vi "PXI-2510 Channel Page.vi"(8 "error in (no error)":errorcluster, 11 "Node Ptr":T2 format="%.0x") -> (0 "error out":errorcluster)   [LabVIEW 2011, in "PXI-2510 Custom Device.lvlib"]
uses:
  PXI-2510 Custom Device.lvlib
  <vilib>/NI Veristand/Custom Device API/Custom Device Item Ref.ctl
  Channel Fault Selector.ctl
  FIU Global Strings.vi
  <vilib>/NI Veristand/Custom Device API/Get Item Property (U16).vi
  <vilib>/NI Veristand/Custom Device API/Custom Device API.lvlib
panel:
  out "Hardware Channel #":u16
  in  "Channel Fault Selector Default Value":T1
  in  "Header":cluster{"Section Name":string}={"Section Name"="Custom Device Item Settings"}
  in  "Description":string
  in  "Name (Alias)":string
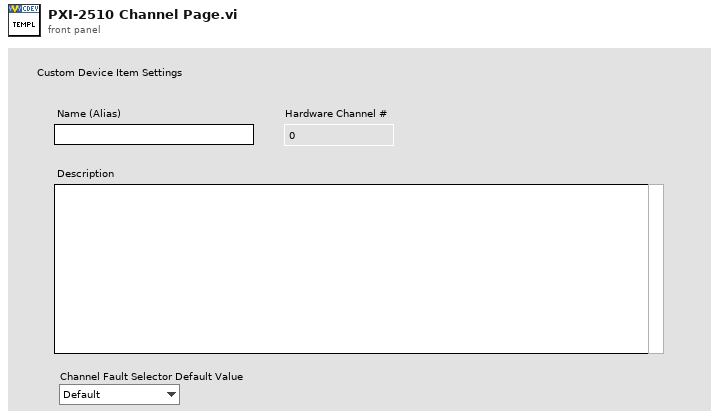
[diagram p1: front panel]
types:
  T1 = typedef "PXI-2510 Custom Device.lvlib/Channel Fault Selector.ctl" = enum16{"Default", "DUT Pass Through", "DUT Open", "DUT Pass Through and FB A", "DUT Pass Through and FB B", "DUT FB A", "DUT FB B"}
  T2 = typedef "Custom Device API.lvlib/Custom Device Item Ref.ctl" = u64
  T3 = typedef "Custom Device API.lvlib/Custom Device Item Info.ctl" = cluster{"Name":string, "Is Channel":bool, "GUID":string}
  T4 = typedef "Custom Device API.lvlib/Custom Device Channel.ctl" = cluster{"Type":T5, "Units":string, "Default Value":dbl, "Faultable":bool, "Scalable":bool}
  T5 = typedef "Custom Device API.lvlib/Custom Device Channel Type.ctl" = enum16{"Input", "Output"}
  T6 = typedef "Custom Device API.lvlib/Custom Device Commands.ctl" = enum16{"Default", "Item renamed", "Shutdown", "Dynamic button pressed"}
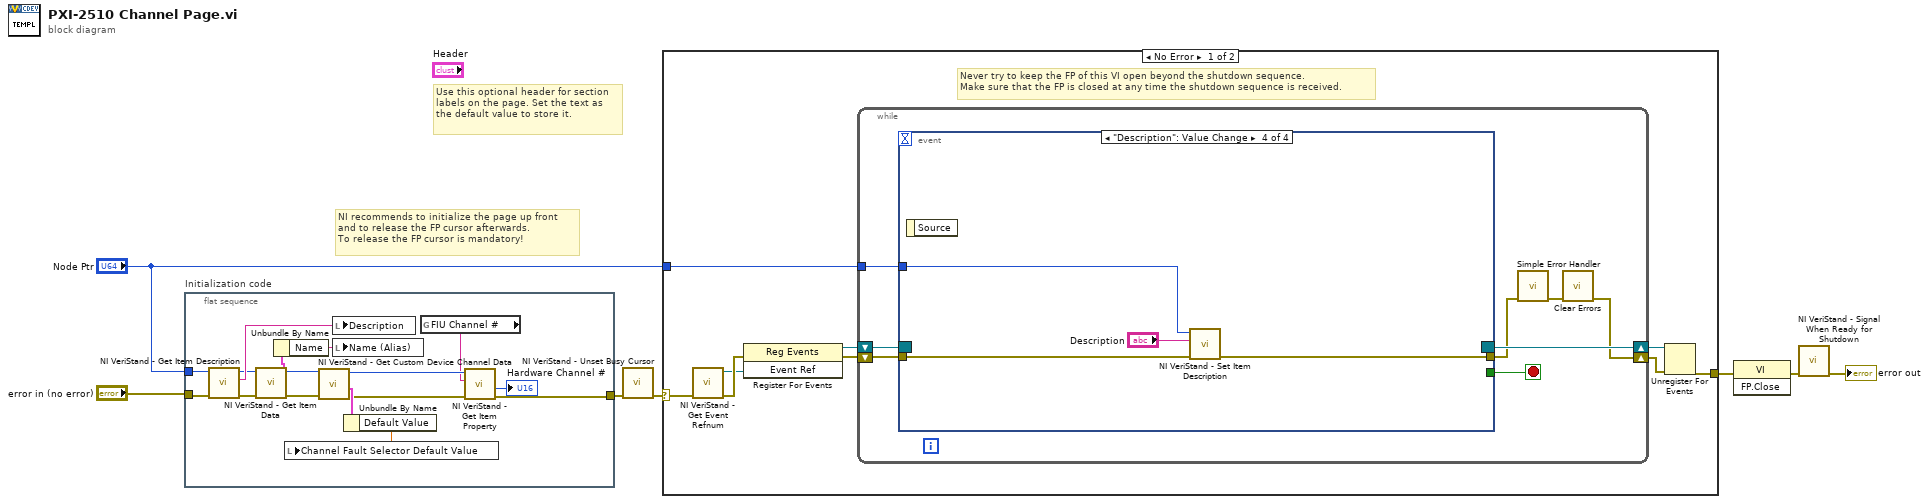
[diagram p0: block diagram]
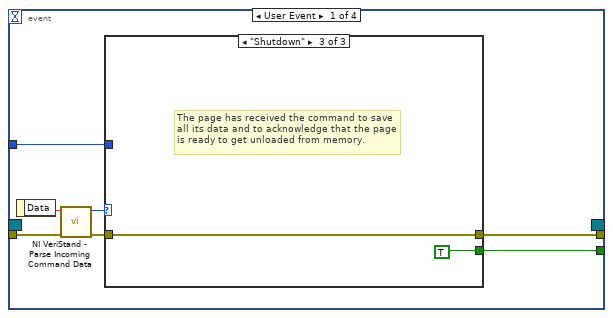
[diagram p2: hidden frame]
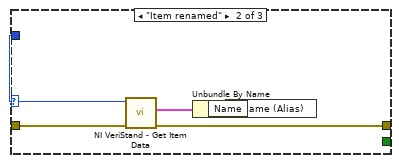
[diagram p4: hidden frame]
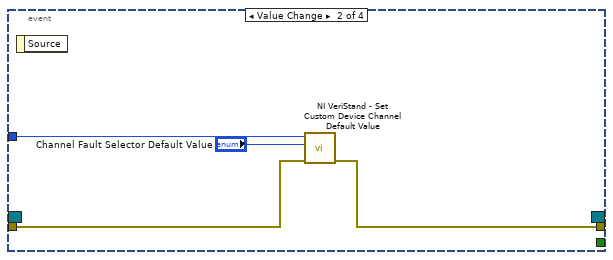
[diagram p5: hidden frame]
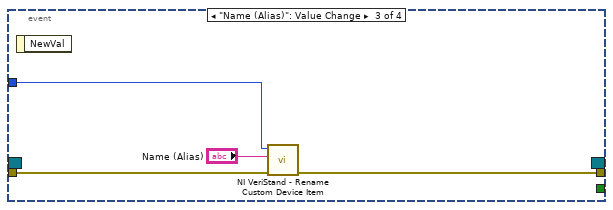
[diagram p6: hidden frame]
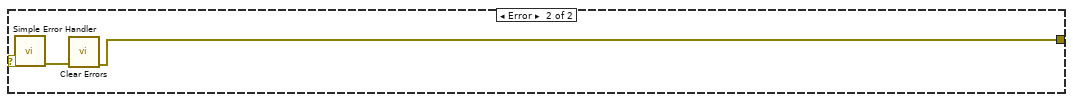
[diagram p7: hidden frame]
diagram:
  # "Use this optional header for section labels on the page. Set the text as the default value to store it."
  # "NI recommends to initialize the page up front\nand to release the FP cursor afterwards.\nTo release the FP cursor is mandatory!"
  n1 = flat-sequence "Initialization code" {
    tunnel: "error in (no error)" -> [w23]
    tunnel: "Node Ptr" -> [w22]
    tunnel: [w8] -> w2
    frame #0 {
      n2 = call <vilib>:"NI VeriStand - Get Item Description.vi"("error in (no error)"=w23, "Item Ref in"=w22) -> ("error out"=w20:errorcluster, "Description"=w21:string, "Item Ref out"=w19:T2)  [unwired: 7 out]
      n3 = call <vilib>:"NI VeriStand - Get Item Data.vi"("error in (no error)"=w20, "Item Ref in"=w19) -> ("error out"=w15:errorcluster, "Item Info"=w18:T3, "Item Ref out"=w16:T2)  [unwired: 7 out]
      n4 = Unbundle By Name(w18) -> ("Name"=w17:string)
      n5 = call <vilib>:"NI VeriStand - Get Custom Device Channel Data.vi"("error in (no error)"=w15, "Channel Ref in"=w16) -> ("error out"=w11:errorcluster, "Channel"=w14:T4, "Channel Ref out"=w12:T2)  [unwired: 4 in, 3 out]
      n6 = local write "Description"(w21) -> ()
      n7 = local write "Name (Alias)"(w17) -> ()
      n8 = Unbundle By Name(w14) -> ("Default Value"=w13:dbl)
      n9 = local write "Channel Fault Selector Default Value"(w13) -> ()
      n10 = global read "FIU Global Strings.vi" "FIU Channel #"() -> (w10:string)
      n11 = call-poly <vilib>:"NI VeriStand - Get Item Property.vi"("error in (no error)"=w11, "Property Name"=w10, "Item Ref in"=w12) -> ("error out"=w8:errorcluster, "Value"=→"Hardware Channel #":u16)  [unwired: 5 in, 2 out]
    }
  }
  n12 = call <vilib>:"NI VeriStand - Unset Busy Cursor.vi"("error in (no error)"=w2) -> ("error out"=w1:errorcluster)  [unwired: 10 out]
  n13 = case shown="No Error" w1 {
    selector: w1 -> [w24 w70]
    tunnel: [w29 w68] -> w5
    tunnel: "Node Ptr" -> [w25 _]
    frame No Error {
      # "Never try to keep the FP of this VI open beyond the shutdown sequence.\nMake sure that the FP is closed at any time the shutdown sequence is received."
      n14 = call <vilib>:"NI VeriStand - Get Event Refnum.vi"("error in (no error)"=w24) -> ("error out"=w32:errorcluster, "Event Ref"=w28:refnum<user-event>)  [unwired: 9 out]
      n15 = register-events(error in=w32, w28) -> (reference out=w26:refnum<event-registration>, error out=w27:errorcluster)  [unwired: 1 in]
      n16 = while {
        tunnel: w25 -> [w36]
        shift-right: [w33] -> w30
        shift-left: w27 -> [w39]
        shift-right: [w40] -> w31
        shift-left: w26 -> [w38]
        stop <- w37 stop-if-true
        n17 = event shown="[3] \"Description\": Value Change" {
          selector: w38 -> [_ _ _ _]
          dyn-events: [_ _ _ _] -> w40
          timeout: _ -> [_ _ _ _]
          tunnel: w39 -> [w47 w57 w63 w66]
          tunnel: [w43 _ _ _] -> w37
          tunnel: [w42 w56 w62 w65] -> w35
          tunnel: w36 -> [w41 w59 w61 w67]
          event User Event {
            n18 = event-data() -> ("Data"=w46:string)  [unwired: 1 out]
            n19 = call <vilib>:"NI VeriStand - Parse Incoming Command Data.vi"("error in (no error)"=w47, "Incoming data"=w46) -> ("error out"=w45:errorcluster, "Action"=w44:T6)  [unwired: 8 out]
            n20 = case shown="\"Shutdown\"" w44 {
              tunnel: w45 -> [w48 w53 w54]
              tunnel: [_ _ TRUE] -> w43
              tunnel: [w48 w50 w54] -> w42
              tunnel: w41 -> [_ w52 _]
              frame "Default", Default {
              }
              frame "Item renamed" {
                n21 = call <vilib>:"NI VeriStand - Get Item Data.vi"("error in (no error)"=w53, "Item Ref in"=w52) -> ("error out"=w50:errorcluster, "Item Info"=w51:T3)  [unwired: 8 out]
                n22 = Unbundle By Name(w51) -> ("Name"=w49:string)
                n23 = local write "Name (Alias)"(w49) -> ()
              }
              frame "Shutdown" {
                # "The page has received the command to save all its data and to acknowledge that the page is ready to get unloaded from memory."
              }
            }
          }
          event Value Change {
            n24 = event-data() -> ()  [unwired: 2 out]
            n25 = call <vilib>:"NI VeriStand - Set Custom Device Channel Default Value.vi"("error in (no error)"=w57, "Default Value"="Channel Fault Selector Default Value", "Channel Ref in"=w59) -> ("error out"=w56:errorcluster)  [unwired: 7 in, 1 out]
          }
          event "Name (Alias)": Value Change {
            n26 = event-data() -> ()  [unwired: 2 out]
            n27 = call <vilib>:"NI VeriStand - Rename Custom Device Item.vi"("error in (no error)"=w63, "New Name"="Name (Alias)", "Item Ref in"=w61) -> ("error out"=w62:errorcluster)  [unwired: 8 out]
          }
          event "Description": Value Change {
            n28 = event-data() -> ()  [unwired: 2 out]
            n29 = call <vilib>:"NI VeriStand - Set Item Description.vi"("error in (no error)"=w66, "Description"="Description", "Item Ref in"=w67) -> ("error out"=w65:errorcluster)  [unwired: 8 out]
          }
        }
        n30 = call <vilib>:"Simple Error Handler.vi"("error in (no error)"=w35) -> ("error out"=w34:errorcluster)  [unwired: 1 in, 7 out]
        n31 = call <vilib>:"Clear Errors.vi"("error in (no error)"=w34) -> ("error out"=w33:errorcluster)  [unwired: 6 out]
      }
      n32 = Unregister For Events(event registration refnum=w31, error in=w30) -> (error out=w29:errorcluster)
    }
    frame Error {
      n33 = call <vilib>:"Simple Error Handler.vi"("error in (no error)"=w70) -> ("error out"=w69:errorcluster)  [unwired: 1 in, 7 out]
      n34 = call <vilib>:"Clear Errors.vi"("error in (no error)"=w69) -> ("error out"=w68:errorcluster)  [unwired: 6 out]
    }
  }
  n35 = invoke class="VI" method="FP.Close"(error in=w5) -> (error out=w4:errorcluster)  [unwired: 2 in, 2 out]
  n36 = call <vilib>:"NI VeriStand - Signal When Ready for Shutdown.vi"("error in (no error)"=w4) -> ("error out"=→"error out":errorcluster)  [unwired: 10 out]
